vi "experiment control.vi"() -> ()   [LabVIEW 2012] (continued)
                n1005 = Enqueue Element At Opposite End(queue=w2495, element="Abort") -> (queue out=w2494:refnum<queue>)  [unwired: 2 in, 2 out]
                n1006 = Enqueue Element At Opposite End(queue=w2494, element="Debug: Popup >> No switches are selected! Aborting.") -> ()  [unwired: 2 in, 3 out]
              }
            }
          }
          frame "Switch: Scan Step" {
            n1007 = Unbundle By Name(w2510) -> ("Switch Scan"=w2507:bool[][], "Switch Scan Index"=w2500:i32)
            n1008 = Multiply(x=100 ("y"), y=w2500) -> (x*y=w2506:i32)
            n1009 = Index Array(array=w2507, index (row)=w2500) -> (element=w2509:bool[])  [unwired: 1 in]
            n1010 = Array To Cluster(array=w2509) -> (cluster=w2508:T91)
            n1011 = Array Size(array=w2507) -> (size(s)=w2504:i32[])
            n1012 = local write "Machine State"(w2508) -> ()
            n1013 = Index Array(array=w2504) -> (element=w2503:i32)  [unwired: 1 in]
            n1014 = Divide(x=w2506, y=w2503) -> (x/y=→"Slide":dbl)
            n1015 = Increment(x=w2500) -> (x+1=w2501:i32)
            n1016 = Bundle By Name(cluster=w2510, "Switch Scan Index"=w2501) -> (w2511:T52)
            n1017 = Enqueue Element At Opposite End(queue=w2498, element="Switch: Set Machine State") -> (queue out=w2499:refnum<queue>)  [unwired: 2 in, 2 out]
          }
          frame "Switch: Set Machine State" {
            n1018 = while {
              shift-right: [w2527] -> _
              shift-left: "Switch: Set >> Brot\nSwitch: Set >> Doublet\nSwitch: Set >> Rotation\nSwitch: Set >> Depletion phase\nSwitch: Set >> Depletion polarization" -> [w2529]
              tunnel: [w2526] -> w2516 mode=indexing
              stop <- w2524 stop-if-true
              n1019 = Match Pattern(string=w2529, regular expression="[\\n\\r]+") -> (before substring=w2526:string, after substring=w2527:string, offset past match=w2525:i32)  [unwired: 1 in, 1 out]
              n1020 = Less Than 0?(x=w2525) -> (x < 0?=w2524:bool)
            }
            n1021 = Reverse 1D Array(array=w2516) -> (reversed array=w2515:string[])
            n1022 = for {
              tunnel: [w2523] -> _
              tunnel: w2514 -> [w2522]
              shift-right: [w2520] -> _
              shift-left: _ -> [w2521]
              tunnel: w2515 -> [w2519] mode=indexing
              n1023 = Enqueue Element At Opposite End(queue=w2522, element=w2519, error in (no error)=w2521) -> (queue out=w2523:refnum<queue>, error out=w2520:errorcluster)  [unwired: 1 in, 1 out]
            }
          }
          frame "Switch: Set" {
            n1024 = local read "Machine State"() -> (w2537:T1)
            n1025 = Match Pattern(string=w2540, regular expression=",") -> (before substring=w2534:string, after substring=w2533:string)  [unwired: 1 in, 2 out]
            n1026 = case shown="\"Doublet\"" w2534 {
              tunnel: w2537 -> [w2552 w2574 w2611 w2628 w2641 _]
              tunnel: "Switch Settings" -> [w2550 w2572 w2609 w2630 _ _]
              tunnel: [w2544 w2565 "Trap DDS: Upload" ("State(s) in Front (\"\")") "Depletion Agilent: Set" ("State(s) in Front (\"\")") w2638 ""] -> w2531
              tunnel: [w2546 w2566 w2603 w2626 w2640 w2642] -> w2538
              tunnel: w2539 -> [w2546 w2566 w2603 w2626 w2640 w2642]
              tunnel: w2533 -> [w2547 _ _ _ _ _]
              frame "Brot" {
                n1027 = Unbundle By Name(w2552) -> ("Brot"=w2551:bool)
                n1028 = Unbundle By Name(w2550) -> ("Brot"=w2549:cluster{"in":dbl, "out":dbl})
                n1029 = Empty String/Path?(string/path=w2547) -> (empty?=w2548:bool)
                n1030 = case shown="True" w2548 {
                  tunnel: w2551 -> [_ w2557]
                  tunnel: [w2553 w2556] -> w2543
                  tunnel: w2549 -> [_ w2555]
                  tunnel: w2547 -> [w2554 _]
                  frame False {
                    n1031 = Fract/Exp String To Number(string=w2554) -> (number=w2553:dbl)  [unwired: 3 in, 1 out]
                  }
                  frame True {
                    n1032 = case shown="False" w2557 {
                      tunnel: w2555 -> [w2559 w2561]
                      tunnel: [w2558 w2560] -> w2556
                      frame True {
                        n1033 = Unbundle By Name(w2559) -> ("in"=w2558:dbl)
                      }
                      frame False {
                        n1034 = Unbundle By Name(w2561) -> ("out"=w2560:dbl)
                      }
                    }
                  }
                }
                n1035 = Number To Exponential String(number=w2543) -> (E-format string=w2542:string)  [unwired: 3 in]
                n1036 = Concatenate Strings("Coils: Set >> Bias,axgrad," ("State(s) in Front (\"\")"), w2542) -> (w2544:string)
              }
              frame "Doublet" {
                n1037 = Unbundle By Name(w2572) -> ("Doublet"=w2571:T92)
                n1038 = Unbundle By Name(w2574) -> ("Doublet"=w2573:bool)
                n1039 = case shown="False" w2573 {
                  tunnel: w2571 -> [w2598 w2602]
                  tunnel: [w2597 w2601] -> w2568
                  tunnel: [w2596 w2600] -> w2567
                  tunnel: [w2595 w2599] -> w2562
                  frame True {
                    n1040 = Unbundle By Name(w2598) -> ("Upper T"=w2595:dbl, "upper"=w2597:dbl, "DurationUpper"=w2596:dbl)
                  }
                  frame False {
                    n1041 = Unbundle By Name(w2602) -> ("Lower T"=w2599:dbl, "lower"=w2601:dbl, "DurationLower"=w2600:dbl)
                  }
                }
                n1042 = local read "DIO64"() -> (w2563:T3)
                n1043 = for {
                  tunnel: w2563 -> [w2579] mode=indexing
                  tunnel: [w2578] -> w2564 mode=indexing
                  tunnel: w2567 -> [w2577]
                  tunnel: w2562 -> [w2575]
                  n1044 = Unbundle By Name(w2579) -> ("Task"=w2576:string)
                  n1045 = case shown="\"Pi/2 Pulse 2\"" w2576 {
                    tunnel: w2579 -> [w2580 w2583 w2587 w2590]
                    tunnel: [w2580 w2582 w2586 w2589] -> w2578
                    tunnel: w2577 -> [_ w2581 w2585 _]
                    tunnel: w2575 -> [_ _ w2584 w2588]
                    frame "False", Default {
                    }
                    frame "Pi/2 Pulse" {
                      n1046 = Bundle By Name(cluster=w2583, "end time"=w2581) -> (w2582:T93)
                    }
                    frame "Pi/2 Pulse 2" {
                      n1047 = Bundle By Name(cluster=w2587, "begin time"=w2584, "end time"=w2585) -> (w2586:T93)
                    }
                    frame "Trigger Depletion 2" {
                      n1048 = disable-structure shown="Enabled" {
                        disable-tunnel: w2590 -> [w2593 w2594]
                        disable-tunnel: [w2592 w2594] -> w2589
                        disable-tunnel: w2588 -> [w2591 _]
                        frame Disabled {
                          n1049 = Bundle By Name(cluster=w2593, "begin time"=w2591) -> (w2592:T93)
                        }
                        frame Enabled {
                        }
                      }
                    }
                  }
                }
                n1050 = Number To Fractional String(number=w2568) -> (F-format string=w2570:string)  [unwired: 3 in]
                n1051 = local write "DIO64"(w2564) -> ()
                n1052 = Concatenate Strings("DDS: Goto Frequency >> 2," ("State(s) in Front (\"\")"), w2570) -> (w2565:string)
              }
              frame "Rotation" {
                n1053 = Unbundle By Name(w2609) -> ("Rotation"=w2608:T94)
                n1054 = Unbundle By Name(w2611) -> ("Rotation"=w2610:bool)
                n1055 = case shown="False" w2610 {
                  tunnel: w2608 -> [w2613 w2615]
                  tunnel: [w2612 w2614] -> w2605
                  frame True {
                    n1056 = Unbundle By Name(w2613) -> ("Down"=w2612:T95)
                  }
                  frame False {
                    n1057 = Unbundle By Name(w2615) -> ("Up"=w2614:T95)
                  }
                }
                n1058 = local read "Trap DDS"() -> (w2607:T26)
                n1059 = Bundle By Name(cluster=w2607, "channels"=w2605) -> (w2606:T26)
                n1060 = local write "Trap DDS"(w2606) -> ()
              }
              frame "Depletion phase" {
                n1061 = Unbundle By Name(w2630) -> ("Depletion phase"=w2629:cluster{"0 phase":dbl, "pi phase":dbl})
                n1062 = Unbundle By Name(w2628) -> ("Depletion phase"=w2627:bool)
                n1063 = case shown="True" w2627 {
                  tunnel: w2629 -> [w2631 w2633]
                  tunnel: [w2632 w2634] -> w2622
                  frame True {
                    n1064 = Unbundle By Name(w2631) -> ("pi phase"=w2632:dbl)
                  }
                  frame False {
                    n1065 = Unbundle By Name(w2633) -> ("0 phase"=w2634:dbl)
                  }
                }
                n1066 = local read "Depletion Agilent"() -> (w2625:T14)
                n1067 = Unbundle By Name(w2625) -> ("Channels"=w2621:T96)
                n1068 = Index Array(array=w2621, index=0) -> (element=w2623:T97)
                n1069 = Bundle By Name(cluster=w2623, "Phase"=w2622) -> (w2620:T97)
                n1070 = Replace Array Subset(array=w2621, new element=w2620, index=0) -> (w2618:T96)
                n1071 = Bundle By Name(cluster=w2625, "Channels"=w2618) -> (w2624:T14)
                n1072 = local write "Depletion Agilent"(w2624) -> ()
              }
              frame "Depletion polarization" {
                n1073 = Unbundle By Name(w2641) -> ("Depletion pol"=w2637:bool)
                n1074 = Boolean To (0,1)(Boolean=w2637) -> (0, 1=w2636:i16)
                n1075 = Number To Decimal String(number=w2636) -> (decimal integer string=w2635:string)  [unwired: 1 in]
                n1076 = Concatenate Strings("Depletion Flip >> " ("State(s) in Front (\"\")"), w2635) -> (w2638:string)
              }
              frame Default {
              }
            }
            n1077 = Enqueue Element At Opposite End(queue=w2530, element=w2531) -> (queue out=w2532:refnum<queue>)  [unwired: 2 in, 2 out]
          }
          frame "Switch: Change State" {
            n1078 = Match Pattern(string=w2664, regular expression=",") -> (before substring=w2659:string, after substring=w2655:string)  [unwired: 1 in, 2 out]
            n1079 = Decimal String To Number(string=w2655) -> (number=w2657:i32)  [unwired: 2 in, 1 out]
            n1080 = local read "Machine State"() -> (w2658:T1)
            n1081 = Not Equal To 0?(x=w2657) -> (x != 0?=w2656:bool)
            n1082 = case shown="\"Depletion phase\"" w2659 {
              tunnel: w2658 -> [w2679 w2683 w2686 w2689 w2692 w2693]
              tunnel: [w2678 w2682 w2685 w2688 w2691 w2693] -> w2649
              tunnel: w2656 -> [w2680 w2681 w2684 w2687 w2690 _]
              frame "Brot" {
                n1083 = Bundle By Name(cluster=w2679, "Brot"=w2680) -> (w2678:T1)
              }
              frame "Doublet" {
                n1084 = Bundle By Name(cluster=w2683, "Doublet"=w2681) -> (w2682:T1)
              }
              frame "Rotation" {
                n1085 = Bundle By Name(cluster=w2686, "Rotation"=w2684) -> (w2685:T1)
              }
              frame "Depletion phase" {
                n1086 = Bundle By Name(cluster=w2689, "Depletion phase"=w2687) -> (w2688:T1)
              }
              frame "Depletion pol" {
                n1087 = Bundle By Name(cluster=w2692, "Depletion pol"=w2690) -> (w2691:T1)
              }
              frame Default {
              }
            }
            n1088 = property on="State Hierarchy" class="LstBox (strict)"() -> ("Item Symbols"=w2648:i32[], "Value"=w2647:i32[])  [unwired: 2 in, 2 out]
            n1089 = for {
              tunnel: w2647 -> [w2667] mode=indexing
              tunnel: w2648 -> [w2666]
              tunnel: [w2665] -> w2654 mode=indexing
              n1090 = Index Array(array=w2666, index=w2667) -> (element=w2665:i32)
            }
            n1091 = local write "Machine State"(w2649) -> ()
            n1092 = Array Size(array=w2654) -> (size(s)=w2653:i32)
            n1093 = Scale By Power Of 2(n=w2653, x=1) -> (x*2^n=w2651:i32)
            n1094 = for {
              N: w2651 -> [_]
              tunnel: w2654 -> [w2671]
              tunnel: w2649 -> [w2669]
              tunnel: [w2668] -> w2650 mode=indexing
              i -> [w2673]
              n1095 = Cluster To Array(cluster=w2669) -> (array=w2670:bool[])
              n1096 = Number To Boolean Array(number=w2673) -> (Boolean array=w2672:bool[])
              n1097 = for {
                tunnel: w2672 -> [w2675] mode=indexing
                tunnel: w2671 -> [w2676] mode=indexing
                shift-right: [w2674] -> w2668
                shift-left: w2670 -> [w2677]
                n1098 = Replace Array Subset(array=w2677, new element=w2675, index=w2676) -> (w2674:bool[])
              }
            }
            n1099 = Bundle By Name(cluster=w2662, "Switch Scan"=w2650) -> (w2661:T52)
            n1100 = Enqueue Element At Opposite End(queue=w2645, element="Switch: Set Machine State") -> (queue out=w2646:refnum<queue>)  [unwired: 2 in, 2 out]
          }
          frame "Switch: Update Hierarchy" {
            n1101 = property on="State Hierarchy" class="LstBox (strict)"() -> ("Item Symbols"=w2701:i32[], "Value"=w2700:i32[])  [unwired: 2 in, 2 out]
            n1102 = local read "Machine State"() -> (w2699:T1)
            n1103 = for {
              tunnel: w2700 -> [w2708] mode=indexing
              tunnel: w2701 -> [w2707]
              tunnel: [w2706] -> w2702 mode=indexing
              n1104 = Index Array(array=w2707, index=w2708) -> (element=w2706:i32)
            }
            n1105 = Array Size(array=w2702) -> (size(s)=w2698:i32)
            n1106 = Scale By Power Of 2(n=w2698, x=1) -> (x*2^n=w2696:i32)
            n1107 = for {
              N: w2696 -> [_]
              tunnel: w2702 -> [w2712]
              tunnel: w2699 -> [w2710]
              tunnel: [w2709] -> w2694 mode=indexing
              i -> [w2714]
              n1108 = Cluster To Array(cluster=w2710) -> (array=w2711:bool[])
              n1109 = Number To Boolean Array(number=w2714) -> (Boolean array=w2713:bool[])
              n1110 = for {
                tunnel: w2713 -> [w2716] mode=indexing
                tunnel: w2712 -> [w2717] mode=indexing
                shift-right: [w2715] -> w2709
                shift-left: w2711 -> [w2718]
                n1111 = Replace Array Subset(array=w2718, new element=w2716, index=w2717) -> (w2715:bool[])
              }
            }
            n1112 = Bundle By Name(cluster=w2704, "Switch Scan"=w2694) -> (w2703:T52)
          }
          frame "---------- Scan ----------" {
            # "Template Separator\n(You can make a copy of, or modify, this frame)"
          }
          frame "Scan: Step" {
            n1113 = Decimal String To Number(string=w2735) -> (number=w2724:i32)  [unwired: 2 in, 1 out]
            n1114 = local read "Scan Variables"() -> (w2728:T32)
            n1115 = Index Array(array=w2728, index=w2724) -> (element=w2727:T98)
            n1116 = Unbundle By Name(w2727) -> ("randomize"=w2723:bool, "scan string"=w2732:string)
            n1117 = local read "Scan References"() -> (w2733:T33)
            n1118 = call "matlab_string_to_array.vi"("String"=w2732) -> ("Array"=w2731:dbl[])  [unwired: 10 in]
            n1119 = case shown="True" w2723 {
              tunnel: w2731 -> [w2739 w2742]
              tunnel: [w2739 w2741] -> w2729
              tunnel: 0.0 -> [_ w2740]
              frame False {
              }
              frame True {
                n1120 = call-poly <vilib>:"Riffle (obs 2012).vi"("seed"=w2740, "X"=w2742) -> ("Riffled {X}"=w2741:dbl[])  [unwired: 7 in, 2 out]
              }
            }
            n1121 = Delete From Array(array=w2729) -> (deleted portion=w2730:dbl)  [unwired: 2 in, 1 out]
            n1122 = Build Array (concatenate)(w2729, w2730) -> (w2726:dbl[])
            n1123 = for {
              tunnel: w2733 -> [w2749] mode=indexing
              tunnel: [w2748] -> w2734 mode=indexing
              shift-right: [w2746] -> w2736
              shift-left: w2737 -> [w2745]
              tunnel: w2726 -> [w2747]
              tunnel: w2722 -> [w2743]
              n1124 = Unbundle By Name(w2749) -> ("scan"=w2750:bool)
              n1125 = case shown="True" w2750 {
                tunnel: w2749 -> [w2752 w2784]
                tunnel: [w2752 w2783] -> w2748
                tunnel: [_ w2773] -> w2744
                tunnel: w2747 -> [_ w2765]
                tunnel: [w2751 w2767] -> w2746
                tunnel: w2745 -> [w2751 w2766]
                frame False {
                }
                frame True {
                  n1126 = Unbundle By Name(w2784) -> ("Reference"=w2770:string, "equation"=w2772:string, "index"=w2758:i32, "next"=w2753:dbl)
                  n1127 = Increment(x=w2758) -> (x+1=w2764:i32)
                  n1128 = call <vilib>:"Eval Single-Variable Array.vi"("error in (no error)"=w2766, "X Values"=w2765, "formula"=w2772) -> ("error out"=w2767:errorcluster, "Y Values"=w2760:dbl[])
                  n1129 = Array Size(array=w2760) -> (size(s)=w2781:i32)
                  n1130 = Less Than 0?(x=w2758) -> (x < 0?=w2755:bool)
                  n1131 = Decrement(x=w2781) -> (x-1=w2761:i32)
                  n1132 = Match Pattern(string=w2770, regular expression=" ") -> (before substring=w2769:string, after substring=w2768:string)  [unwired: 1 in, 2 out]
                  n1133 = In Range and Coerce(upper limit=w2761, x=w2764, lower limit=0) -> (coerced(x)=w2774:i32)  [unwired: 1 out]
                  n1134 = Index Array(array=w2760, index=w2774) -> (element=w2756:dbl)
                  n1135 = Select(t=w2756, s=w2755, f=w2753) -> (s? t:f=w2757:dbl)
                  n1136 = case shown="\"Stella\"" w2769 {
                    tunnel: w2757 -> [_ w2787 w2790 w2794 w2808 w2822 w2836 w2846 w2858 w2878 w2886]
                    tunnel: [_ _ _ _ _ _ w2835 _ w2857 _ w2888] -> w2773
                    tunnel: w2768 -> [_ _ _ w2791 w2805 w2819 w2833 w2847 w2859 w2879 _]
                    frame Default {
                    }
                    frame "Stella" {
                      n1137 = local read "Stella"() -> (w2785:T20)
                      n1138 = Bundle By Name(cluster=w2785, "setpoint"=w2787) -> (w2786:T20)
                      n1139 = local write "Stella"(w2786) -> ()
                    }
                    frame "Jessica" {
                      n1140 = local read "Jessica"() -> (w2788:T17)
                      n1141 = Bundle By Name(cluster=w2788, "setpoint"=w2790) -> (w2789:T17)
                      n1142 = local write "Jessica"(w2789) -> ()
                    }
                    frame "End" {
                      n1143 = local read "DIO64"() -> (w2793:T3)
                      n1144 = for {
                        tunnel: w2793 -> [w2798] mode=indexing
                        tunnel: w2791 -> [w2800]
                        tunnel: w2794 -> [w2797]
                        tunnel: [w2796] -> w2792 mode=indexing
                        n1145 = Unbundle By Name(w2798) -> ("Task"=w2799:string)
                        n1146 = Equal?(x=w2799, y=w2800) -> (x = y?=w2795:bool)
                        n1147 = case shown="True" w2795 {
                          tunnel: w2798 -> [w2801 w2804]
                          tunnel: w2797 -> [_ w2803]
                          tunnel: [w2801 w2802] -> w2796
                          frame False {
                          }
                          frame True {
                            n1148 = Bundle By Name(cluster=w2804, "end time"=w2803) -> (w2802:T93)
                          }
                        }
                      }
                      n1149 = local write "DIO64"(w2792) -> ()
                    }
                    frame "Begin" {
                      n1150 = local read "DIO64"() -> (w2807:T3)
                      n1151 = for {
                        tunnel: w2807 -> [w2812] mode=indexing
                        tunnel: w2805 -> [w2814]
                        tunnel: w2808 -> [w2811]
                        tunnel: [w2810] -> w2806 mode=indexing
                        n1152 = Unbundle By Name(w2812) -> ("Task"=w2813:string)
                        n1153 = Equal?(x=w2813, y=w2814) -> (x = y?=w2809:bool)
                        n1154 = case shown="True" w2809 {
                          tunnel: w2812 -> [w2815 w2818]
                          tunnel: w2811 -> [_ w2817]
                          tunnel: [w2815 w2816] -> w2810
                          frame False {
                          }
                          frame True {
                            n1155 = Bundle By Name(cluster=w2818, "begin time"=w2817) -> (w2816:T93)
                          }
                        }
                      }
                      n1156 = local write "DIO64"(w2806) -> ()
                    }
                    frame "DAC" {
                      n1157 = local read "DAC Schedule"() -> (w2821:T6)
                      n1158 = for {
                        tunnel: w2821 -> [w2826] mode=indexing
                        tunnel: w2819 -> [w2828]
                        tunnel: w2822 -> [w2825]
                        tunnel: [w2824] -> w2820 mode=indexing
                        n1159 = Unbundle By Name(w2826) -> ("Task"=w2827:string)
                        n1160 = Equal?(x=w2827, y=w2828) -> (x = y?=w2823:bool)
                        n1161 = case shown="True" w2823 {
                          tunnel: w2826 -> [w2829 w2832]
                          tunnel: w2825 -> [_ w2831]
                          tunnel: [w2829 w2830] -> w2824
                          frame False {
                          }
                          frame True {
                            n1162 = Bundle By Name(cluster=w2832, "Begin"=w2831) -> (w2830:T99)
                          }
                        }
                      }
                      n1163 = local write "DAC Schedule"(w2820) -> ()
                    }
                    frame "DDS" {
                      n1164 = case shown="\"Channel 1\", Default" w2833 {
                        tunnel: [1 2 3 4] -> w2834
                        frame "Channel 1", Default {
                        }
                        frame "Channel 2" {
                        }
                        frame "Channel 3" {
                        }
                        frame "Channel 4" {
                        }
                      }
                      n1165 = Number To Decimal String(number=w2834) -> (decimal integer string=w2839:string)  [unwired: 1 in]
                      n1166 = Number To Exponential String(number=w2836, precision (6)=i16 9) -> (E-format string=w2838:string)  [unwired: 2 in]
                      n1167 = Concatenate Strings("DDS: Goto Frequency >> " ("string"), w2839, "," ("string"), w2838) -> (w2835:string)
                    }
                    frame "Trap" {
                      # "\"Trap DDS Frequency\""
                      n1168 = case shown="\"DDS Frequency\", Default" w2847 {
                        tunnel: w2846 -> [w2848]
                        frame "DDS Frequency", Default {
                          n1169 = local read "Trap DDS"() -> (w2851:T26)
                          n1170 = Unbundle By Name(w2851) -> ("channels"=w2852:T95)
                          n1171 = for {
                            tunnel: w2852 -> [w2855] mode=indexing
                            tunnel: [w2854] -> w2850 mode=indexing
                            tunnel: w2848 -> [w2853]
                            n1172 = Bundle By Name(cluster=w2855, "Frequency"=w2853) -> (w2854:T100)
                          }
                          n1173 = Bundle By Name(cluster=w2851, "channels"=w2850) -> (w2849:T26)
                          n1174 = local write "Trap DDS"(w2849) -> ()
                        }
                      }
                    }
                    frame "Microwave" {
                      n1175 = case shown="\"Power\"" w2859 {
                        tunnel: w2858 -> [w2867 w2871 w2875]
                        tunnel: [TRUE TRUE FALSE] -> w2856
                        frame "Begin", Default {
                          n1176 = local read "HP8341B"() -> (w2868:T27)
                          n1177 = Bundle By Name(cluster=w2868, "frequency"=w2867) -> (w2869:T27)
                          n1178 = local write "HP8341B"(w2869) -> ()
                        }
                        frame "End" {
                          n1179 = local read "HP8341B"() -> (w2872:T27)
                          n1180 = Bundle By Name(cluster=w2872, "stop frequency"=w2871) -> (w2873:T27)
                          n1181 = local write "HP8341B"(w2873) -> ()
                        }
                        frame "Power" {
                          n1182 = local read "HP8341B"() -> (w2876:T27)
                          n1183 = Bundle By Name(cluster=w2876, "power"=w2875) -> (w2877:T27)
                          n1184 = local write "HP8341B"(w2877) -> ()
                        }
                      }
                      n1185 = case shown="False" w2856 {
                        tunnel: ["Microwave: Set Power" w2863] -> w2857
                        frame False {
                        }
                        frame True {
                          n1186 = local read "HP8341B"() -> (w2862:T27)
                          n1187 = Unbundle By Name(w2862) -> ("Chirp"=w2861:bool)
                          n1188 = case shown="True" w2861 {
                            tunnel: ["Microwave: Set Sweep" "Microwave: Set Frequency"] -> w2863
                            frame True {
                            }
                            frame False {
                            }
                          }
                        }
                      }
                    }
                    frame "Doublet" {
                      n1189 = case shown="\"Upper T\", Default" w2879 {
                        tunnel: w2878 -> [w2880 w2883]
                        frame "Upper T", Default {
                          n1190 = local read "Switch Settings"() -> (w2881:T9)
                          n1191 = Bundle By Name(cluster=w2881, "Doublet.Upper T"=w2880) -> (w2882:T9)
                          n1192 = local write "Switch Settings"(w2882) -> ()
                        }
                        frame "Lower T" {
                          n1193 = local read "Switch Settings"() -> (w2884:T9)
                          n1194 = Bundle By Name(cluster=w2884, "Doublet.Lower T"=w2883) -> (w2885:T9)
                          n1195 = local write "Switch Settings"(w2885) -> ()
                        }
                      }
                    }
                    frame "Brot" {
                      n1196 = Number To Fractional String(number=w2886) -> (F-format string=w2887:string)  [unwired: 3 in]
                      n1197 = Concatenate Strings("Switch: Set >> Brot,", w2887) -> (w2888:string)
                    }
                  }
                  n1198 = Increment(x=w2764) -> (x+1=w2763:i32)
                  n1199 = In Range and Coerce(upper limit=w2761, x=w2763, lower limit=0) -> (coerced(x)=w2759:i32)  [unwired: 1 out]
                  n1200 = Index Array(array=w2760, index=w2759) -> (element=w2754:dbl)
                  n1201 = To Double Precision Float(number=w2774) -> (double precision float=w2776:dbl)
                  n1202 = To Double Precision Float(number=w2761) -> (double precision float=w2775:dbl)
                  n1203 = Divide(x=w2776, y=w2775) -> (x/y=w2778:dbl)
                  n1204 = Multiply(x=w2778, y=100.0) -> (x*y=w2777:dbl)
                  n1205 = To Unsigned Byte Integer(number=w2777) -> (unsigned 8bit integer=w2780:u8)
                  n1206 = Bundle By Name(cluster=w2784, "next"=w2754, "index"=w2774, "progress"=w2780) -> (w2783:T57)
                }
              }
              n1207 = Enqueue Element At Opposite End(queue=w2743, element=w2744) -> ()  [unwired: 2 in, 3 out]
            }
            n1208 = local write "Scan References"(w2734) -> ()
          }
          frame "Scan: Reset" {
            n1209 = Decimal String To Number(string=w2897) -> (number=w2894:i32)  [unwired: 2 in, 1 out]
            n1210 = Number To Decimal String(number=w2894) -> (decimal integer string=w2892:string)  [unwired: 1 in]
            n1211 = local read "Scan References"() -> (w2895:T33)
            n1212 = for {
              tunnel: w2895 -> [w2901] mode=indexing
              tunnel: [w2900] -> w2896 mode=indexing
              n1213 = Unbundle By Name(w2901) -> ("scan"=w2902:bool)
              n1214 = case shown="True" w2902 {
                tunnel: w2901 -> [w2903 w2906]
                tunnel: [w2903 w2905] -> w2900
                frame False {
                }
                frame True {
                  n1215 = Bundle By Name(cluster=w2906, "index"=-1) -> (w2905:T57)
                }
              }
            }
            n1216 = Concatenate Strings("Scan: Step >> ", w2892) -> (w2891:string)
            n1217 = Enqueue Element At Opposite End(queue=w2890, element=w2891) -> ()  [unwired: 2 in, 3 out]
            n1218 = local write "Scan References"(w2896) -> ()
          }
          frame "Scan: Reference" {
            n1219 = Match Pattern(string=w2912, regular expression=",") -> (before substring=w2909:string, after substring=w2907:string)  [unwired: 1 in, 2 out]
            n1220 = case shown="\"Disable\", Default" w2909 {
              tunnel: [FALSE TRUE] -> w2908
              frame "Disable", Default {
              }
              frame "Enable" {
              }
            }
            n1221 = case shown="\"0\", Default" w2907 {
              tunnel: w2907 -> [w2917 _]
              tunnel: w2908 -> [w2915 _]
              frame "0", Default {
                n1222 = local read "Scan References"() -> (w2920:T33)
                n1223 = Decimal String To Number(string=w2917) -> (number=w2916:i32)  [unwired: 2 in, 1 out]
                n1224 = Index Array(array=w2920, index=w2916) -> (element=w2921:T57)
                n1225 = Bundle By Name(cluster=w2921, "scan"=w2915) -> (w2919:T57)
                n1226 = Replace Array Subset(array=w2920, new element=w2919, index=w2916) -> (w2918:T33)
                n1227 = local write "Scan References"(w2918) -> ()
              }
              frame "All" {
                n1228 = local read "Scan References"() -> (w2923:T33)
                n1229 = for {
                  tunnel: w2923 -> [w2926] mode=indexing
                  tunnel: [w2925] -> w2922 mode=indexing
                  n1230 = Bundle By Name(cluster=w2926, "scan"=FALSE) -> (w2925:T57)
                }
                n1231 = local write "Scan References"(w2922) -> ()
              }
            }
          }
          frame "---------- Lasers ----------" {
            # "Template Separator\n(You can make a copy of, or modify, this frame)"
          }
          frame "Laser: Step Wavelength" {
            n1232 = case shown="Default" w2935 {
              tunnel: w2934 -> [w2937 w2941 w2999 w3053 w3086]
              tunnel: [w2937 w2940 w2998 w3053 w3086] -> w2933
              tunnel: w2932 -> [_ _ _ w3052 w3085]
              frame Default {
              }
              frame "TiSapph" {
                n1233 = local read "TiSapph"() -> (w2942:T18)
                n1234 = Unbundle By Name(w2942) -> ("setpoint"=w2938:dbl, "Channel"=w2939:tag, "scan"=w2943:bool)
                n1235 = case shown="True" w2943 {
                  tunnel: w2942 -> [_ w2953]
                  tunnel: w2941 -> [w2944 w2951]
                  tunnel: [w2944 w2950] -> w2940
                  tunnel: w2939 -> [_ w2949]
                  tunnel: w2938 -> [_ w2947]
                  frame False {
                  }
                  frame True {
                    n1236 = Unbundle By Name(w2953) -> ("scan start"=w2957:dbl, "scan end"=w2956:dbl, "scan step"=w2971:dbl, "scan start"=w2973:dbl, "scan end"=w2972:dbl, "scan step"=w2969:dbl, "setpoint"=w2968:dbl, "scan start"=w2958:dbl, "scan end"=w2959:dbl)
                    n1237 = Less?(x=w2973, y=w2972) -> (x < y?=w2974:bool)
                    n1238 = Negate(x=w2969) -> (-x=w2970:dbl)
                    n1239 = Subtract(x=w2959, y=w2958) -> (x-y=w2965:dbl)
                    n1240 = Select(t=w2971, s=w2974, f=w2970) -> (s? t:f=w2967:dbl)
                    n1241 = Add(x=w2967, y=w2968) -> (x+y=w2952:dbl)
                    n1242 = Max & Min(x=w2957, y=w2956) -> (max(x,y)=w2955:dbl, min(x,y)=w2954:dbl)
                    n1243 = Subtract(x=w2952, y=w2958) -> (x-y=w2966:dbl)
                    n1244 = In Range and Coerce(upper limit=w2955, x=w2952, lower limit=w2954) -> (coerced(x)=w2945:dbl)  [unwired: 1 out]
                    n1245 = Divide(x=w2966, y=w2965) -> (x/y=w2964:dbl)
                    n1246 = Subtract(x=w2945, y=w2947) -> (x-y=w2948:dbl)
                    n1247 = Multiply(x=100.0, y=w2964) -> (x*y=w2962:dbl)
                    n1248 = Sign(1:w2948) -> (0:w2946:dbl)
                    n1249 = To Unsigned Byte Integer(number=w2962) -> (unsigned 8bit integer=w2961:u8)
                    n1250 = while {
                      tunnel: w2951 -> [w2988]
                      tunnel: [w2987] -> w2950
                      tunnel: w2949 -> [w2986]
                      shift-right: [w2975] -> _
                      shift-left: w2947 -> [w2977]
                      tunnel: w2946 -> [w2980]
                      tunnel: w2945 -> [w2979]
                      stop <- w2978 stop-if-true
                      n1251 = Multiply(x=w2980, y=0.001) -> (x*y=w2984:dbl)
                      n1252 = call-poly <vilib>:"DAQmx Create Virtual Channel.vi"("maximum value"=10.0, "minimum value"=0.0, "physical channels"=w2986, "error in"=w2988) -> ("task out"=w2996:refnum<k21>, "error out"=w2995:errorcluster)  [unwired: 10 in]
                      n1253 = Add(x=w2977, y=w2984) -> (x+y=w2983:dbl)
                      n1254 = Max & Min(x=w2977, y=w2979) -> (max(x,y)=w2982:dbl, min(x,y)=w2981:dbl)
                      n1255 = In Range and Coerce(upper limit=w2982, x=w2983, lower limit=w2981) -> (coerced(x)=w2975:dbl)  [unwired: 1 out]
                      n1256 = call-poly <vilib>:"DAQmx Write.vi"("task/channels in"=w2996, "data"=w2975, "error in"=w2995) -> ("task out"=w2992:refnum<k21>, "error out"=w2997:errorcluster)  [unwired: 10 in, 1 out]
                      n1257 = Equal?(x=w2975, y=w2979) -> (x = y?=w2978:bool)
                      n1258 = call <vilib>:"DAQmx Start Task.vi"("task/channels in"=w2992, "error in"=w2997) -> ("task out"=w2991:refnum<k21>, "error out"=w2990:errorcluster)  [unwired: 12 in]
                      n1259 = call <vilib>:"DAQmx Clear Task.vi"("task in"=w2991, "error in"=w2990) -> ("error out"=w2989:errorcluster)  [unwired: 13 in]
                      n1260 = call "wait.vi"("error in (no error)"=w2989, "ms to wait"=u32 5) -> ("error out (no error)"=w2987:errorcluster)  [unwired: 7 in]
                    }
                    n1261 = Bundle By Name(cluster=w2953, "setpoint"=w2945, "progress"=w2961) -> (w2960:T18)
                    n1262 = local write "TiSapph"(w2960) -> ()
                  }
                }
              }
              frame "Stella" {
                n1263 = local read "Stella"() -> (w3001:T20)
                n1264 = Unbundle By Name(w3001) -> ("scan"=w3000:bool)
                n1265 = case shown="True" w3000 {
                  tunnel: w3001 -> [_ w3006]
                  tunnel: w2999 -> [w3002 w3004]
                  tunnel: [w3002 w3003] -> w2998
                  frame False {
                  }
                  frame True {
                    n1266 = Tick Count (ms)() -> (millisecond timer value=w3005:u32)
                    n1267 = stacked-sequence {
                      seq-local: [w3008 _] -> [_ w3034]
                      seq-local: [w3007 _] -> [_ w3033]
                      tunnel: w3006 -> [w3009 _]
                      tunnel: w3005 -> [_ w3035]
                      tunnel: w3004 -> [w3007 _]
                      tunnel: [_ w3032] -> w3003
                      frame #0 {
                        n1268 = Unbundle By Name(w3009) -> ("scan start"=w3015:dbl, "scan end"=w3014:dbl, "scan step"=w3028:dbl, "scan start"=w3030:dbl, "scan end"=w3029:dbl, "scan step"=w3026:dbl, "setpoint"=w3025:dbl, "scan start"=w3016:dbl, "scan end"=w3017:dbl)
                        n1269 = Less?(x=w3030, y=w3029) -> (x < y?=w3031:bool)
                        n1270 = Negate(x=w3026) -> (-x=w3027:dbl)
                        n1271 = Subtract(x=w3017, y=w3016) -> (x-y=w3022:dbl)
                        n1272 = Select(t=w3028, s=w3031, f=w3027) -> (s? t:f=w3024:dbl)
                        n1273 = Add(x=w3024, y=w3025) -> (x+y=w3011:dbl)
                        n1274 = Max & Min(x=w3015, y=w3014) -> (max(x,y)=w3013:dbl, min(x,y)=w3012:dbl)
                        n1275 = In Range and Coerce(upper limit=w3013, x=w3011, lower limit=w3012) -> (coerced(x)=w3010:dbl)  [unwired: 1 out]
                        n1276 = Subtract(x=w3010, y=w3016) -> (x-y=w3023:dbl)
                        n1277 = Divide(x=w3023, y=w3022) -> (x/y=w3021:dbl)
                        n1278 = Multiply(x=100.0, y=w3021) -> (x*y=w3019:dbl)
                        n1279 = To Unsigned Byte Integer(number=w3019) -> (unsigned 8bit integer=w3018:u8)
                        n1280 = Bundle By Name(cluster=w3009, "setpoint"=w3010, "progress"=w3018) -> (w3008:T20)
                        n1281 = local write "Stella"(w3008) -> ()
                      }
                      frame #1 {
                        n1282 = while {
                          tunnel: w3034 -> [w3051]
                          tunnel: w3035 -> [w3046]
                          shift-right: [w3037] -> w3032
                          shift-left: w3033 -> [w3037]
                          stop <- w3041 stop-if-true
                          n1283 = Unbundle By Name(w3051) -> ("wavelength"=w3036:dbl, "setpoint"=w3040:dbl, "lock tolerance"=w3048:dbl)
                          n1284 = Subtract(x=w3036, y=w3040) -> (x-y=w3050:dbl)
                          n1285 = Absolute Value(x=w3050) -> (abs(x)=w3049:dbl)
                          n1286 = Less?(x=w3049, y=w3048) -> (x < y?=w3042:bool)
                          n1287 = local read "Stella"() -> (w3038:T20)
                          n1288 = Bundle By Name(cluster=w3038, "wavelength"=w3036) -> (w3039:T20)
                          n1289 = Tick Count (ms)() -> (millisecond timer value=w3047:u32)
                          n1290 = Subtract(x=w3047, y=w3046) -> (x-y=w3045:u32)
                          n1291 = Greater?(x=w3045, y=u32 10000) -> (0:w3043:bool)
                          n1292 = local write "Stella"(w3039) -> ()
                          n1293 = Or(x=w3042, y=w3043) -> (x .or. y?=w3041:bool)
                        }
                      }
                    }
                  }
                }
              }
              frame "Cora" {
                n1294 = local read "Cora"() -> (w3055:T21)
                n1295 = Unbundle By Name(w3055) -> ("scan"=w3054:bool)
                n1296 = case shown="True" w3054 {
                  tunnel: w3055 -> [_ w3059]
                  tunnel: w3052 -> [_ w3057]
                  frame False {
                  }
                  frame True {
                    n1297 = Unbundle By Name(w3059) -> ("scan start"=w3063:dbl, "scan end"=w3062:dbl, "scan step"=w3077:dbl, "scan start"=w3079:dbl, "scan end"=w3078:dbl, "scan step"=w3075:dbl, "setpoint"=w3074:dbl, "scan start"=w3064:dbl, "scan end"=w3065:dbl)
                    n1298 = Less?(x=w3079, y=w3078) -> (x < y?=w3080:bool)
                    n1299 = Negate(x=w3075) -> (-x=w3076:dbl)
                    n1300 = Subtract(x=w3065, y=w3064) -> (x-y=w3071:dbl)
                    n1301 = Select(t=w3077, s=w3080, f=w3076) -> (s? t:f=w3073:dbl)
                    n1302 = Add(x=w3073, y=w3074) -> (x+y=w3058:dbl)
                    n1303 = Max & Min(x=w3063, y=w3062) -> (max(x,y)=w3061:dbl, min(x,y)=w3060:dbl)
                    n1304 = In Range and Coerce(upper limit=w3061, x=w3058, lower limit=w3060) -> (In Range?=w3056:bool)  [unwired: 1 out]
                    n1305 = Subtract(x=w3058, y=w3064) -> (x-y=w3072:dbl)
                    n1306 = case shown="True" w3056 {
                      tunnel: w3057 -> [_ w3083]
                      frame False {
                      }
                      frame True {
                        n1307 = Enqueue Element At Opposite End(queue=w3083, element="Wait >> 1000" ("t")) -> (queue out=w3084:refnum<queue>)  [unwired: 2 in, 2 out]
                        n1308 = Enqueue Element At Opposite End(queue=w3084, element="DIO64: Trigger >> A8" ("t")) -> ()  [unwired: 2 in, 3 out]
                      }
                    }
                    n1309 = Divide(x=w3072, y=w3071) -> (x/y=w3070:dbl)
                    n1310 = Multiply(x=100.0, y=w3070) -> (x*y=w3068:dbl)
                    n1311 = To Unsigned Byte Integer(number=w3068) -> (unsigned 8bit integer=w3067:u8)
                    n1312 = Bundle By Name(cluster=w3059, "setpoint"=w3058, "progress"=w3067) -> (w3066:T21)
                    n1313 = local write "Cora"(w3066) -> ()
                  }
                }
              }
              frame "Bertha" {
                n1314 = local read "Bertha"() -> (w3088:T22)
                n1315 = Unbundle By Name(w3088) -> ("scan"=w3087:bool)
                n1316 = case shown="True" w3087 {
                  tunnel: w3088 -> [_ w3092]
                  tunnel: w3085 -> [_ w3090]
                  frame False {
                  }
                  frame True {
                    n1317 = Unbundle By Name(w3092) -> ("scan start"=w3096:dbl, "scan end"=w3095:dbl, "scan step"=w3110:dbl, "scan start"=w3112:dbl, "scan end"=w3111:dbl, "scan step"=w3108:dbl, "setpoint"=w3107:dbl, "scan start"=w3097:dbl, "scan end"=w3098:dbl)
                    n1318 = Less?(x=w3112, y=w3111) -> (x < y?=w3113:bool)
                    n1319 = Negate(x=w3108) -> (-x=w3109:dbl)
                    n1320 = Subtract(x=w3098, y=w3097) -> (x-y=w3104:dbl)
                    n1321 = Select(t=w3110, s=w3113, f=w3109) -> (s? t:f=w3106:dbl)
                    n1322 = Add(x=w3106, y=w3107) -> (x+y=w3091:dbl)
                    n1323 = Max & Min(x=w3096, y=w3095) -> (max(x,y)=w3094:dbl, min(x,y)=w3093:dbl)
                    n1324 = In Range and Coerce(upper limit=w3094, x=w3091, lower limit=w3093) -> (In Range?=w3089:bool)  [unwired: 1 out]
                    n1325 = Subtract(x=w3091, y=w3097) -> (x-y=w3105:dbl)
                    n1326 = case shown="True" w3089 {
                      tunnel: w3090 -> [_ w3116]
                      frame False {
                      }
                      frame True {
                        n1327 = Enqueue Element At Opposite End(queue=w3116, element="Wait >> 1000" ("t")) -> (queue out=w3117:refnum<queue>)  [unwired: 2 in, 2 out]
                        n1328 = Enqueue Element At Opposite End(queue=w3117, element="DIO64: Trigger >> C9" ("t")) -> ()  [unwired: 2 in, 3 out]
                      }
                    }
                    n1329 = Divide(x=w3105, y=w3104) -> (x/y=w3103:dbl)
                    n1330 = Multiply(x=100.0, y=w3103) -> (x*y=w3101:dbl)
                    n1331 = To Unsigned Byte Integer(number=w3101) -> (unsigned 8bit integer=w3100:u8)
                    n1332 = Bundle By Name(cluster=w3092, "setpoint"=w3091, "progress"=w3100) -> (w3099:T22)
                    n1333 = local write "Bertha"(w3099) -> ()
                  }
                }
              }
            }
          }
          frame "Laser: Start Scan" {
            n1334 = case shown="\"TiSapph\"" w3121 {
              tunnel: w3120 -> [w3123 w3124 w3158 w3192 w3225 w3230]
              tunnel: [w3123 w3125 w3157 w3191 w3225 w3230] -> w3119
              frame Default {
              }
              frame "TiSapph" {
                n1335 = local read "TiSapph"() -> (w3133:T18)
                n1336 = Unbundle By Name(w3133) -> ("Channel"=w3130:tag, "scan start"=w3126:dbl, "setpoint"=w3129:dbl)
                n1337 = Bundle By Name(cluster=w3133, "setpoint"=w3126, "progress"=u8 0 ("number")) -> (w3132:T18)
                n1338 = local write "TiSapph"(w3132) -> ()
                n1339 = Subtract(x=w3126, y=w3129) -> (x-y=w3128:dbl)
                n1340 = Sign(1:w3128) -> (0:w3127:dbl)
                n1341 = while {
                  tunnel: [w3147] -> w3125
                  tunnel: w3130 -> [w3146]
                  shift-right: [w3137] -> _
                  shift-left: w3126 -> [w3139]
                  tunnel: w3127 -> [w3136]
                  tunnel: w3126 -> [w3134]
